vi "Display Biometry WTW Image.vi"(8 "错误常量":errorcluster, 9 "L_Or_R":string, 10 "Measure_No":i32, 11 "connection reference":T2) -> (0 "error out":errorcluster)   [LabVIEW 2015, in "Browse.lvlib"]
uses:
  Browse.lvlib
  <vilib>/addons/database/Connection.llb/Conn ObjectReference.ctl
  Support/Display Biometry Image State.ctl
  Support/Biometry Image UI Data.ctl
  Sub VIs/Database Processing/Database Processing.lvlib
  <vilib>/addons/database/NI_Database_API.lvlib
  Sub VIs/Utility VIs/Utility VIs.lvlib
panel:
  out "Parameter":string[][](table)
  out "Image 5":T1(plugin-control)
  out "Image 4":T1(plugin-control)
  out "Image 3":T1(plugin-control)
  out "Image 2":T1(plugin-control)
  out "Image":T1(plugin-control)
  in  "停止按钮":bool
  out "状态栏":string
  # "眼睛图像参数"
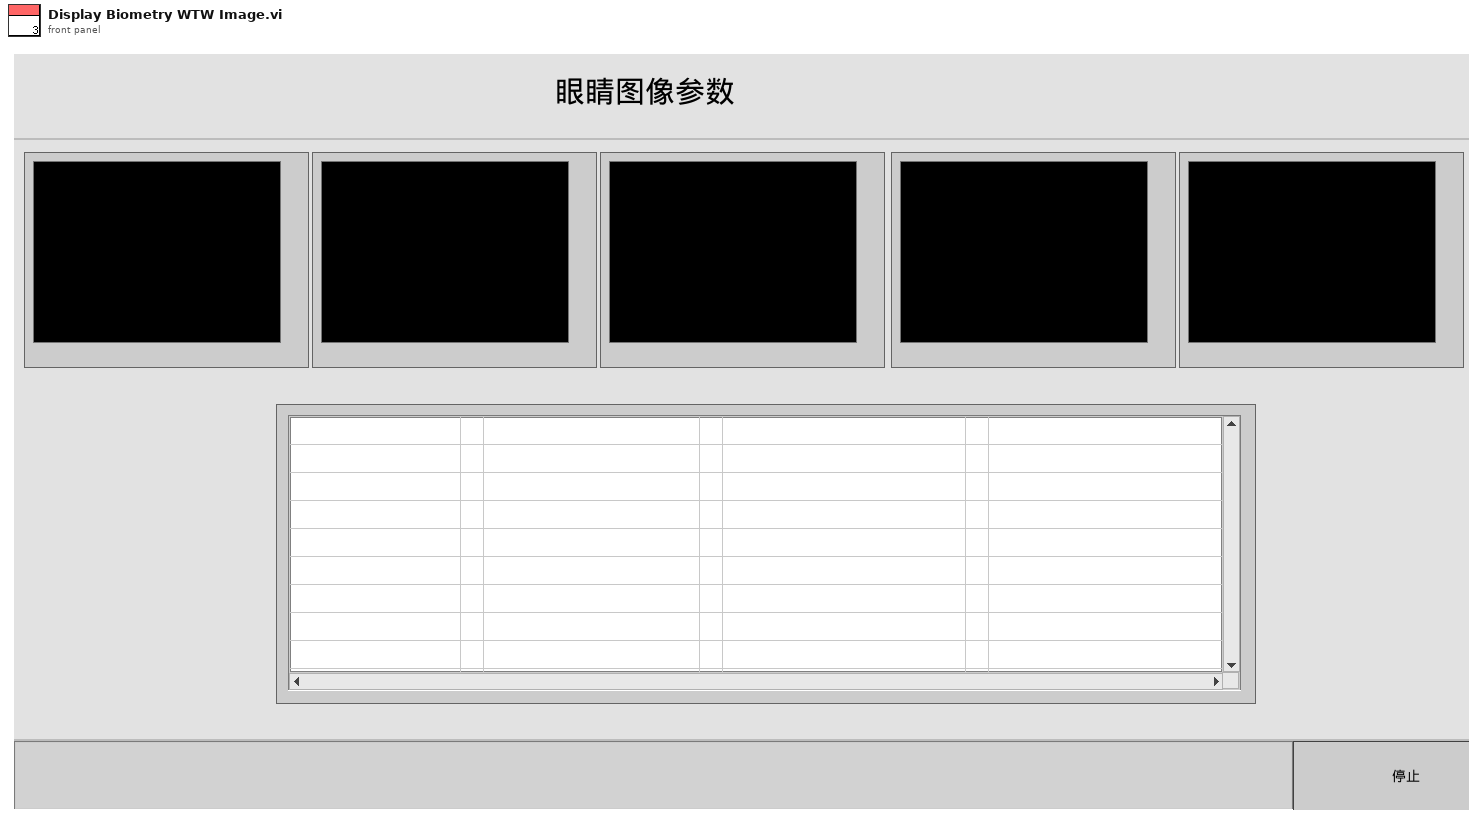
[diagram p1: front panel]
types:
  T1 = typedef "IMAQ Image.ctl" = refnum<image>
  T2 = typedef "NI_Database_API.lvlib/Conn ObjectReference.ctl" = refnum<k1>
  T3 = typedef "Browse.lvlib/Biometry Image UI Data.ctl" = cluster{"Parameter引用句柄":refnum<vi>, "状态栏引用句柄":refnum<vi>, "退出引用句柄":refnum<vi>}
  T4 = typedef "Browse.lvlib/Display Biometry Image State.ctl" = enum16{"Initialize", "Connect Database", "Update Biometry Image", "Update Biometry Image Parameter", "Wait For Event", "Exit"}
  T5 = typedef "LVPoint32TypeDef.ctl" = cluster{"Horizontal":i32, "Vertical":i32}
  T6 = typedef "LVRowAndColumnTypeDef.ctl" = cluster{"Row":i32, "Column":i32}
  T7 = typedef "Database Processing.lvlib/Biometry Data Path.ctl" = cluster{"Measure_ID":i64, "Ascan_data_Original":string, "picture_pupil_Original":string, "picture_WTW_Original":string, "Ascan_data_Processing":string, "picture_pupil_Processing":string, "picture_WTW_Processing":string, "picture_Processing_K":string, "picture_Processing_ALL":string}
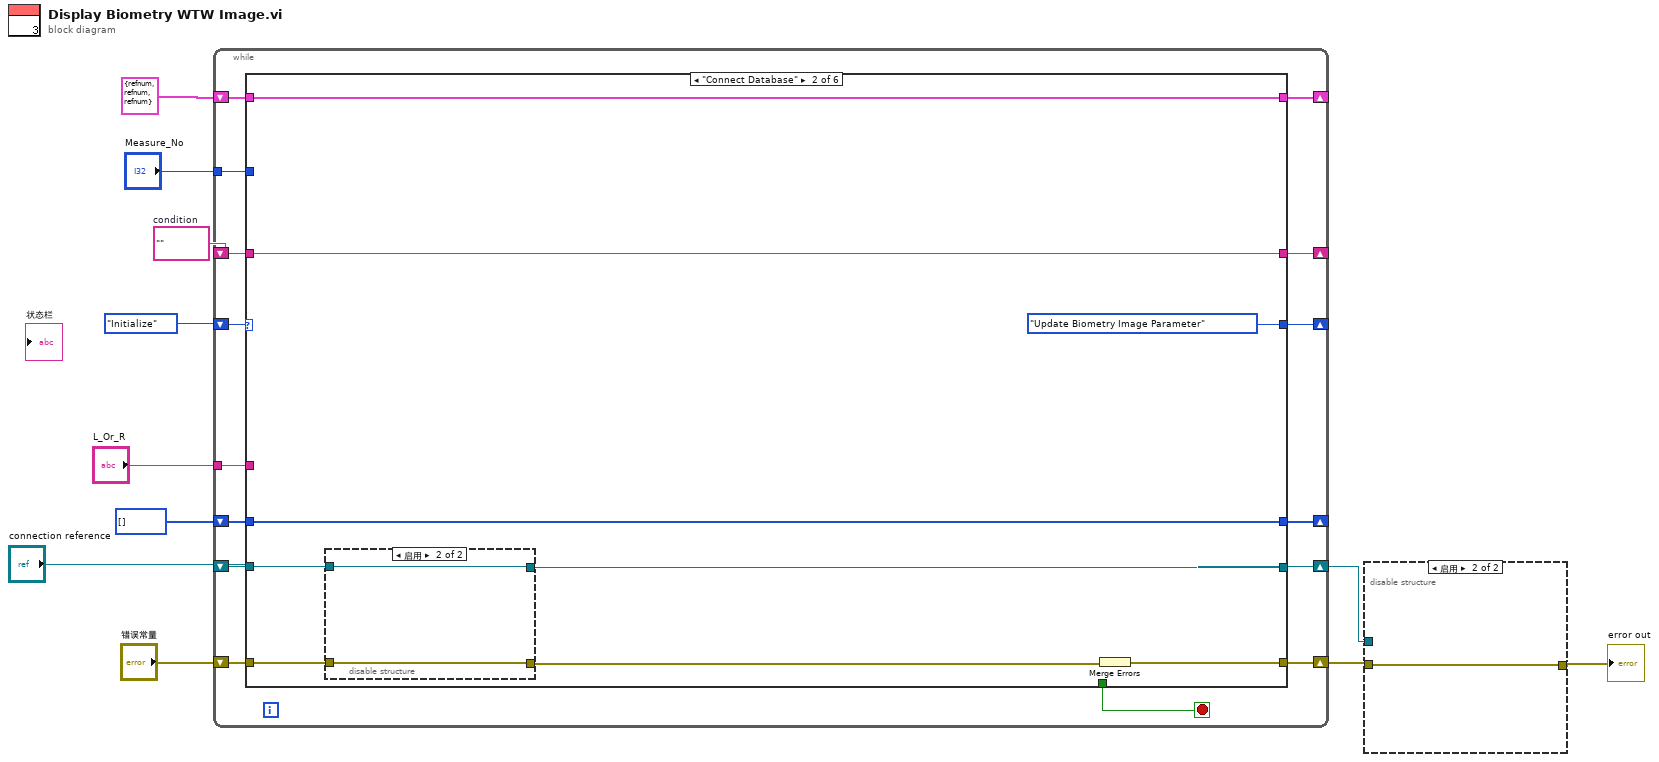
[diagram p0: block diagram]
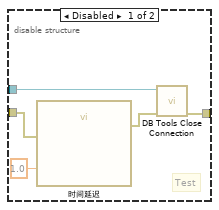
[diagram p2: hidden frame]
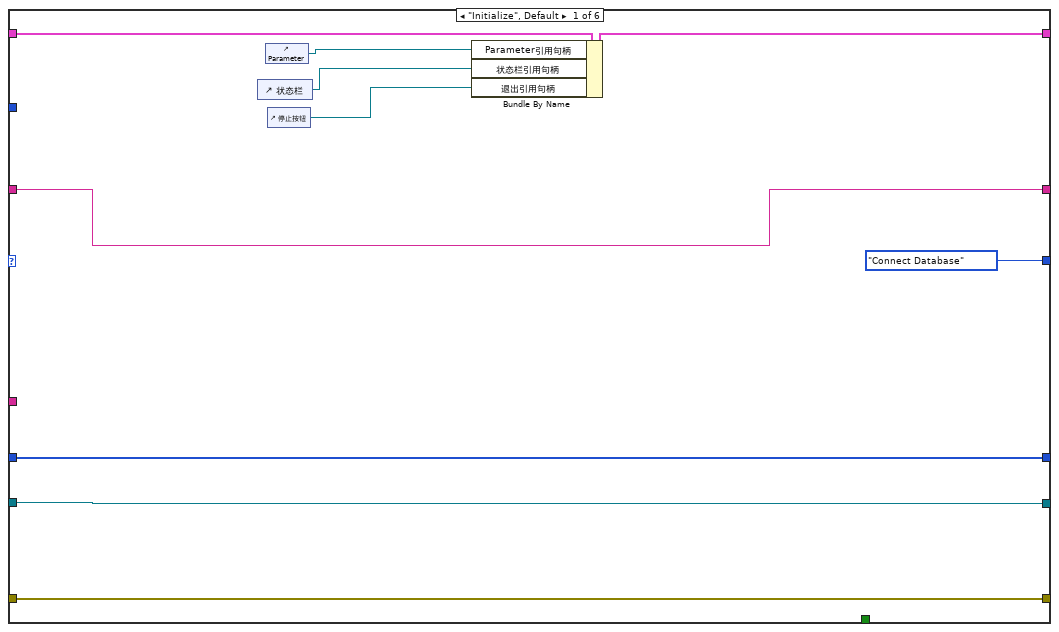
[diagram p3: hidden frame]
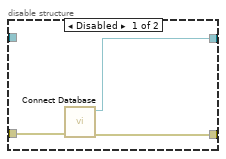
[diagram p4: hidden frame]
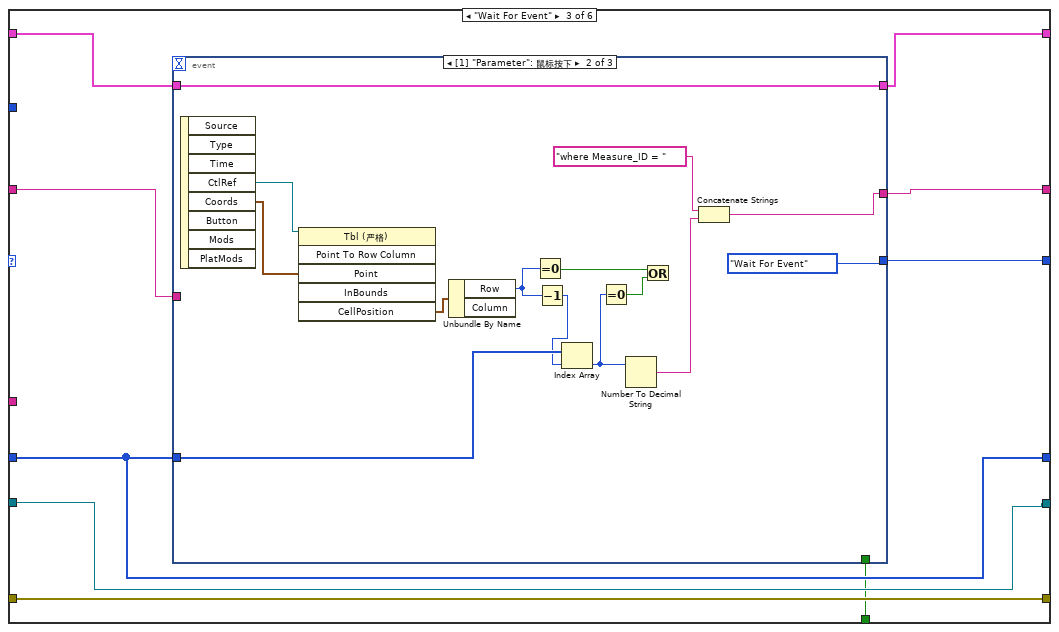
[diagram p5: hidden frame]
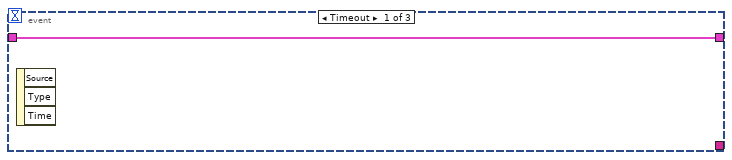
[diagram p6: hidden frame]
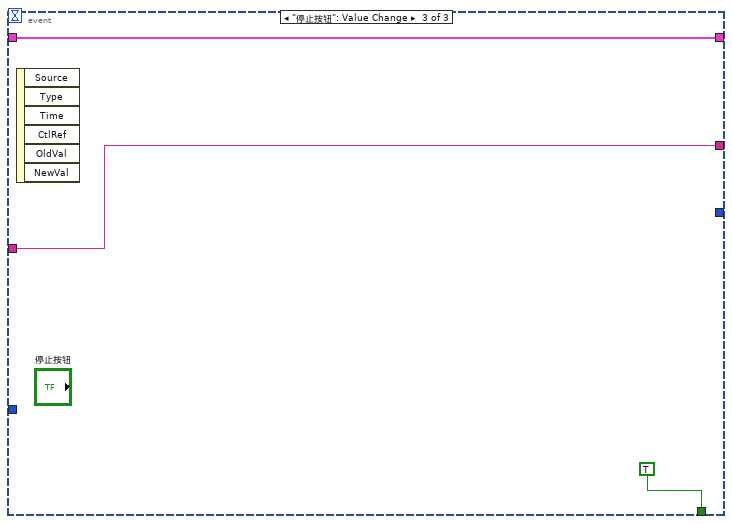
[diagram p7: hidden frame]
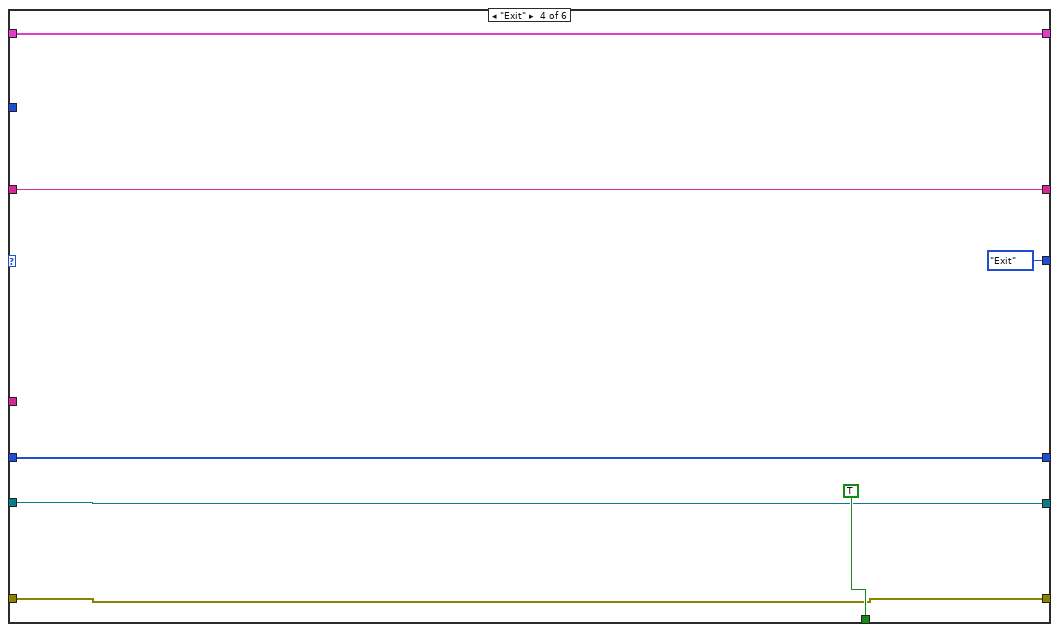
[diagram p8: hidden frame]
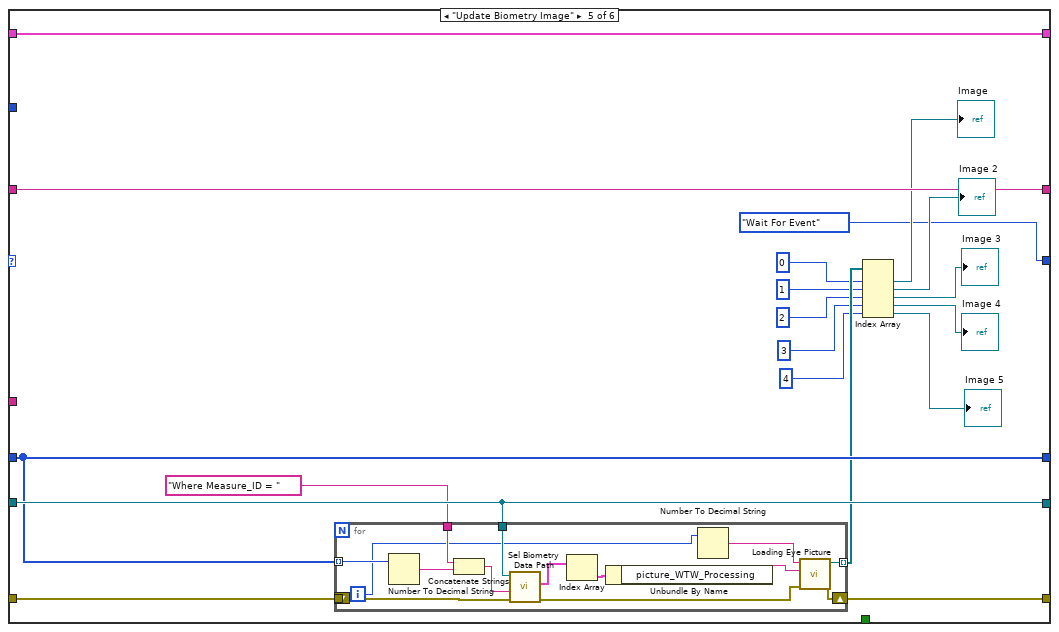
[diagram p9: hidden frame]
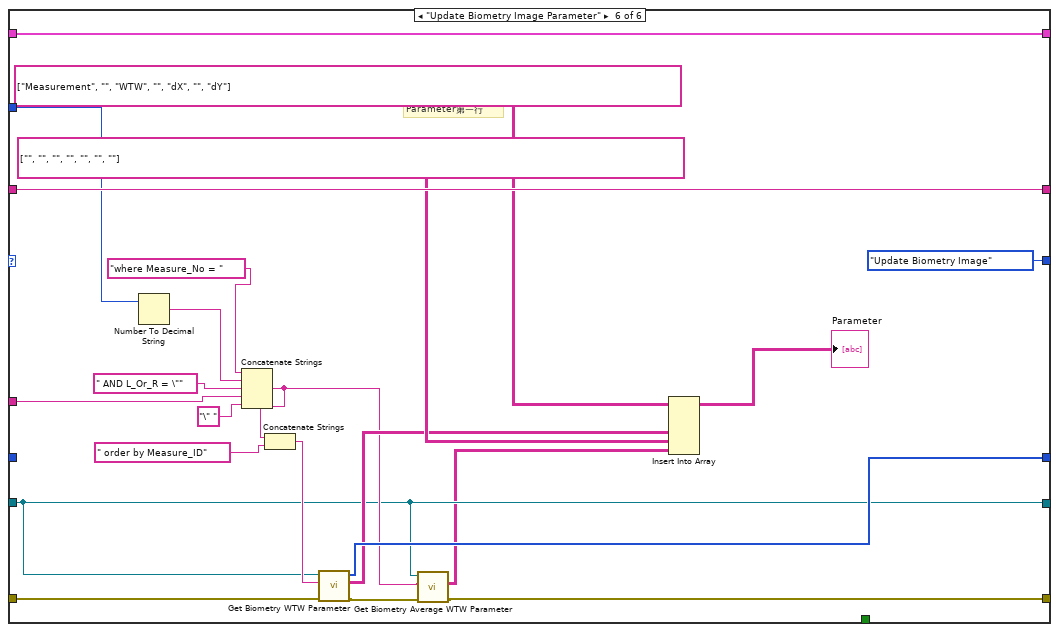
[diagram p10: hidden frame]
diagram:
  w9 = ""  # condition
  n1 = while {
    shift-right: [w25] -> _
    shift-left: T3 {"Parameter引用句柄"=refnum, "状态栏引用句柄"=refnum, "退出引用句柄"=refnum} ("UI数据") -> [w26]
    shift-right: [w17] -> _
    shift-left: Display_Biometry_Image_State."Initialize" ("State") -> [w16]
    shift-right: [w22] -> w5
    shift-left: "错误常量" -> [w24]
    shift-right: [w20] -> _
    shift-left: w9 -> [w23]
    shift-right: [w19] -> w3
    shift-left: "connection reference" -> [w18]
    shift-right: [w15] -> _
    shift-left: i64[] [] -> [w12]
    tunnel: "Measure_No" -> [w14]
    tunnel: "L_Or_R" -> [w13]
    stop <- w21 stop-if-true
    n2 = case shown="\"Connect Database\"" w16 {
      tunnel: w26 -> [w36 w40 w56 w84 w103 w139]
      tunnel: [w35 w40 w55 w84 w103 w139] -> w25
      tunnel: [Display_Biometry_Image_State."Connect Database" ("State") Display_Biometry_Image_State."Update Biometry Image Parameter" ("State") w54 Display_Biometry_Image_State."Exit" ("State") Display_Biometry_Image_State."Wait For Event" ("State") Display_Biometry_Image_State."Update Biometry Image" ("State")] -> w17
      tunnel: w24 -> [w34 w44 w57 w81 w98 w126]
      tunnel: w23 -> [w33 w41 w59 w83 w102 w138]
      tunnel: [w34 w45 w57 w81 w99 w118] -> w22
      tunnel: [w33 w41 w58 w83 w102 w138] -> w20
      tunnel: [_ _ w51 TRUE _ _] -> w21
      tunnel: w18 -> [w32 w38 w52 w80 w101 w120]
      tunnel: [w32 w42 w52 w80 w101 w120] -> w19
      tunnel: [w31 w39 w53 w79 w97 w124] -> w15
      tunnel: w14 -> [_ _ _ _ _ w137]
      tunnel: w13 -> [_ _ _ _ _ w135]
      tunnel: w12 -> [w31 w39 w53 w79 w97 _]
      frame "Initialize", Default {
        n3 = control-ref of="状态栏"() -> (w30:refnum<vi>)
        n4 = control-ref of="Parameter"() -> (w28:refnum<vi>)
        n5 = control-ref of="停止按钮"() -> (w29:refnum<vi>)
        n6 = Bundle By Name(cluster=w36, "Parameter引用句柄"=w28, "状态栏引用句柄"=w30, "退出引用句柄"=w29) -> (w35:T3)
      }
      frame "Connect Database" {
        n7 = disable-structure shown="启用" {
          disable-tunnel: w44 -> [w48 w49]
          disable-tunnel: [w47 w49] -> w43
          disable-tunnel: [w46 w50] -> w42
          disable-tunnel: w38 -> [_ w50]
          frame Disabled {
            n8 = call "Connect Database.vi"("error in (no error)"=w48) -> ("error out"=w47:errorcluster, "connection reference"=w46:T2)  [unwired: 9 in]
          }
          frame Enabled {
          }
        }
        n9 = Merge Errors(w43) -> (w45:errorcluster)
      }
      frame "Wait For Event" {
        n10 = event shown="[1] \"Parameter\": 鼠标按下" {
          selector: _ -> [_ _ _]
          dyn-events: _ -> [_ _ _]
          timeout: _ -> [_ _ _]
          tunnel: w59 -> [_ _ w77]
          tunnel: [_ w71 w77] -> w58
          tunnel: w56 -> [w60 w72 w76]
          tunnel: [w60 w72 w76] -> w55
          tunnel: w53 -> [_ w70 _]
          tunnel: [_ Display_Biometry_Image_State."Wait For Event" ("State") _] -> w54
          tunnel: [_ _ TRUE] -> w51
          event Timeout {
            n11 = event-data() -> ()  [unwired: 1 in, 3 out]
          }
          event "Parameter": Mouse Down {
            n12 = event-data() -> ("CtlRef"=w62:refnum<vi>, "Coords"=w61:T5)  [unwired: 1 in, 6 out]
            n13 = invoke on="调用节点" class="Tbl (严格)" method="Point To Row Column"(reference=w62, "Point"=w61) -> ("CellPosition"=w74:T6)  [unwired: 4 in, 5 out]
            n14 = Unbundle By Name(w74) -> ("Row"=w68:i32)  [unwired: 1 out]
            n15 = Equal To 0?(x=w68) -> (x = 0?=w64:bool)
            n16 = Decrement(x=w68) -> (x-1=w67:i32)
            n17 = Index Array(array=w70, index=w67) -> (element=w66:i64)
            n18 = Equal To 0?(x=w66) -> (x = 0?=w65:bool)
            n19 = Number To Decimal String(number=w66) -> (decimal integer string=w69:string)  [unwired: 1 in]
            n20 = Or(x=w64, y=w65) -> ()  [unwired: 1 out]
            n21 = Concatenate Strings("where Measure_ID = " ("字符串"), w69) -> (w71:string)
          }
          event "停止按钮": Value Change {
            n22 = event-data() -> ()  [unwired: 1 in, 6 out]
          }
        }
      }
      frame "Exit" {
      }
      frame "Update Biometry Image" {
        n23 = for {
          tunnel: w98 -> [w117]
          tunnel: w101 -> [w116]
          tunnel: w97 -> [w115] mode=indexing
          tunnel: "Where Measure_ID = " ("字符串") -> [w113]
          shift-right: [w107] -> w99
          shift-left: _ -> [_]
          tunnel: [w106] -> w96 mode=indexing
          i -> [w104]
          n24 = Number To Decimal String(number=w115) -> (decimal integer string=w114:string)  [unwired: 1 in]
          n25 = Concatenate Strings(w113, w114) -> (w112:string)
          n26 = call "Sel Biometry Data Path.vi"("error in (no error)"=w117, "condition"=w112, "connection reference"=w116) -> ("error out"=w108:errorcluster, "Biometry Data Path"=w111:T7[])  [unwired: 7 in]
          n27 = Index Array(array=w111) -> (element=w110:T7)  [unwired: 1 in]
          n28 = Unbundle By Name(w110) -> ("picture_WTW_Processing"=w109:string)
          n29 = Number To Decimal String(number=w104) -> (decimal integer string=w105:string)  [unwired: 1 in]
          n30 = call "Loading Eye Picture.vi"("error in (no error)"=w108, "名称或相对路径"=w109, "Image Name"=w105) -> ("error out"=w107:errorcluster, "Image Out"=w106:T1)  [unwired: 7 in]
        }
        n31 = Index Array(array=w96, index #1=0 ("索引"), index #2=1 ("索引"), index #3=2 ("索引"), index #4=3 ("索引"), index #5=4 ("索引")) -> (element #1=→"Image":T1, element #2=→"Image 2":T1, element #3=→"Image 3":T1, element #4=→"Image 4":T1, element #5=→"Image 5":T1)
      }
      frame "Update Biometry Image Parameter" {
        # "Parameter第一行"
        n32 = Number To Decimal String(number=w137) -> (decimal integer string=w134:string)  [unwired: 1 in]
        n33 = Concatenate Strings("where Measure_No = " ("字符串"), w134, " AND L_Or_R = \"" ("字符串"), w135, "\" " ("字符串")) -> (w121:string)
        n34 = Concatenate Strings(w121, " order by Measure_ID" ("字符串")) -> (w125:string)
        n35 = call "Get Biometry WTW Parameter.vi"("error in (no error)"=w126, "condition"=w125, "connection reference"=w120) -> ("error out"=w122:errorcluster, "Data Output"=w123:string[][], "Measure_ID"=w124:i64[])  [unwired: 6 in]
        n36 = call "Get Biometry Average WTW Parameter.vi"("error in (no error)"=w122, "condition"=w121, "connection reference"=w120) -> ("error out"=w118:errorcluster, "Data Output"=w119:string[][])  [unwired: 7 in]
        n37 = Insert Into Array(array=string[][] [["Measurement", "", "WTW", "", "dX", "", "dY"]], new element #1=w123, new element #2=string[][] [["", "", "", "", "", "", ""]], new element #3=w119) -> (→"Parameter":string[][])  [unwired: 2 in]
      }
    }
  }
  n38 = disable-structure shown="启用" {
    disable-tunnel: w5 -> [w142 w145]
    disable-tunnel: [w144 w145] -> w4
    disable-tunnel: w3 -> [w143 _]
    frame Disabled {
      # "Test"
      n39 = call "时间延迟"("error in (no error)"=w142, "Delay Time (s)"=1.0) -> ("error out"=w141:errorcluster)  [unwired: 9 in]
      n40 = call <vilib>:"DB Tools Close Connection.vi"("error in (no error)"=w141, "connection reference"=w143) -> ("error out"=w144:errorcluster)  [unwired: 5 in]
    }
    frame Enabled {
    }
  }
  "error out" <- w4
